vi "Main.vi"() -> ()   [LabVIEW 2020]
panel:
  out "MulOut":dbl
  out "SubOut":dbl
  out "AddOut":dbl
  out "DivOut":dbl
  in  "ALU Inputs":T1
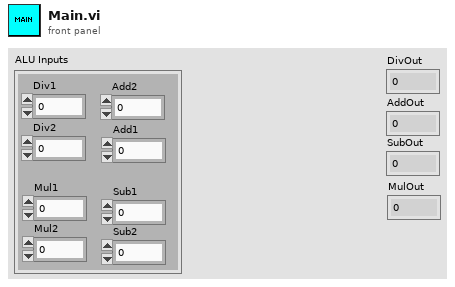
[diagram p1: front panel]
types:
  T1 = cluster{"Div1":dbl, "Div2":dbl, "Add1":dbl, "Add2":dbl, "Sub1":dbl, "Sub2":dbl, "Mul1":dbl, "Mul2":dbl}
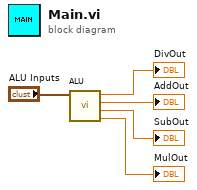
[diagram p0: block diagram]
diagram:
  n1 = call "ALU.vi"("ALU Inputs"="ALU Inputs") -> ("MulOut"=→"MulOut":dbl, "SubOut"=→"SubOut":dbl, "AddOut"=→"AddOut":dbl, "DivOut"=→"DivOut":dbl)  [unwired: 7 in]
